vi "Convert Column to Address.vi"(8 "shift value":i8, 9 "max address":u8, 10 "column(updated)":u8, 11 "address of column zero":u8) -> (3 "address":u8 format="%.0x")   [LabVIEW 2017, in "HD44780.lvclass"]
uses:
  HD44780.lvclass
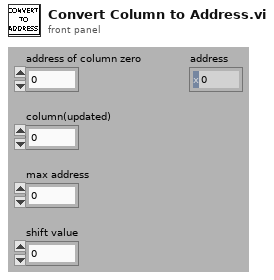
[diagram p1: front panel]
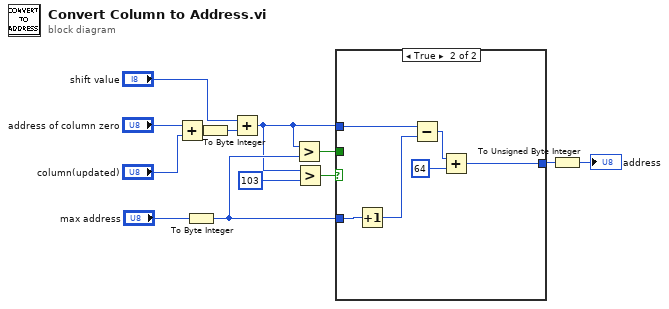
[diagram p0: block diagram]
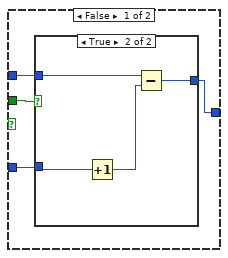
[diagram p2: hidden frame]
diagram:
  n1 = Add(x="address of column zero", y="column(updated)") -> (x+y=w6:u8)
  n2 = To Byte Integer(number="max address") -> (8bit integer=w3:i8)
  n3 = To Byte Integer(number=w6) -> (8bit integer=w5:i8)
  n4 = Add(x="shift value", y=w5) -> (x+y=w2:i8)
  n5 = Greater?(x=w2, y=w3) -> (0:w10:bool)
  n6 = Greater?(x=w2, y=i8 103) -> (0:w7:bool)
  n7 = case shown="True" w7 {
    tunnel: [w17 w23] -> w11
    tunnel: w10 -> [w16 _]
    tunnel: w3 -> [w15 w26]
    tunnel: w2 -> [w14 w27]
    frame False {
      n8 = case shown="True" w16 {
        tunnel: w14 -> [w18 w22]
        tunnel: [w18 w19] -> w17
        tunnel: w15 -> [_ w21]
        frame False {
        }
        frame True {
          n9 = Increment(x=w21) -> (x+1=w20:i8)
          n10 = Subtract(x=w22, y=w20) -> (x-y=w19:i8)
        }
      }
    }
    frame True {
      n11 = Increment(x=w26) -> (x+1=w28:i8)
      n12 = Subtract(x=w27, y=w28) -> (x-y=w25:i8)
      n13 = Add(x=w25, y=i8 64) -> (x+y=w23:i8)
    }
  }
  n14 = To Unsigned Byte Integer(number=w11) -> (unsigned 8bit integer=→"address":u8)
